vi "Data_Save_summary.vi"(6 "ErrorIndex":i32, 8 "Data in":T1, 11 "AllControls In":T2) -> (2 "data":string[](array[string]), 3 "dup path":path)   [LabVIEW 2017]
uses:
  Ctrls/AllControls.ctl
  Ctrls/CSV_Data.ctl
  Ctrls/PathChoose.ctl
  <vilib>/Utility/file.llb/Write Delimited Spreadsheet (string).vi
  <vilib>/Utility/file.llb/Read Delimited Spreadsheet (string).vi
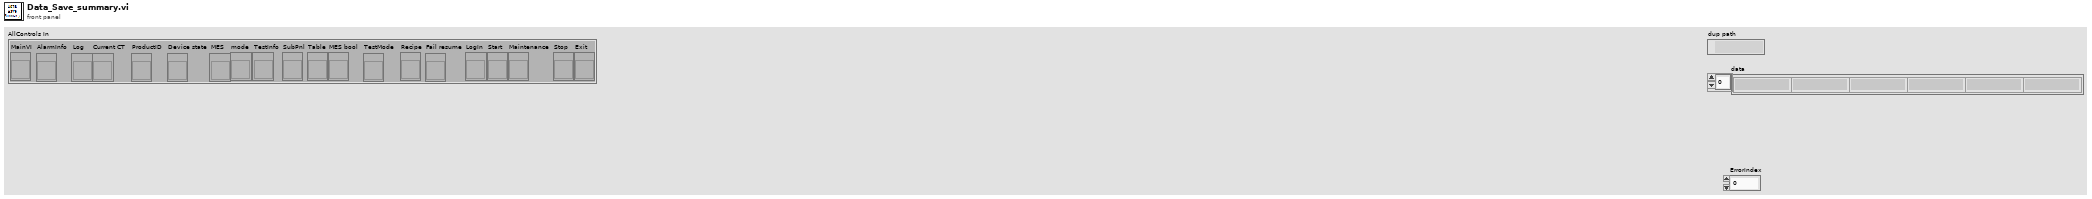
[diagram p1: front panel]
types:
  T1 = typedef "CSV_Data.ctl" = cluster{"Initialisation":cluster{"LMT - Connect UUT (con COM)":string, "LMT - Software Version (rrel)":string, "LMT - Write SKU file (wskuc)":string, "LMT - SKU file name":string, "Connect UUT DDM":string, "Read DDM EOL Timestamp - Mode":string, "Read DDM EOL Timestamp - Timestamp":string, "Read DDM EOL Timestamp - Rig ID":string, "Read DDM EOL Timestamp - Passmark ID":string, "Read DDM EOL Timestamp - Passmark Rev":string, "Software Version before flashing":string, "Read Hardware Serial":string, "UUT DDM SN":string, "Compare DDM SN with MES SN":string, "Backup PCBA Calibration EEPROM Response - CAL":string, "Flash Firmware Version":string, "Check SW Version":string, "Read DDM SW Version after flashing":string, "Set SKU Config":string, "Ready Status":string, "Set Device Mode to EOL":string, "DDM Parameter - Voltage":string, "DDM Parameter - Current":string, "DDM Parameter - Power":string, "DDM Parameter - Speed":string, "DDM Parameter - Pressure":string, "Tester Parameter - Voltage":string, "Tester Parameter - Current":string, "Tester Parameter - Power":string, "Tester Parameter - Ambient Pressure":string, "Tester Parameter - Ambient Temperature":string, "Calculated Parameter - DDM Pressure Corrected":string, "Calculated Parameter - DDM Real Power":string, "Calculated Parameter - Delta V":string}, "BEMF_Calibration":cluster{"Calibration Result - eol_cold_bemf_temp":string, "DDM Ambient Temp":string, "Restriction Plate Diameter":string, "Calibration Result - eol_bemf_mp_cold_coef_a":string, "Calibration Result - eol_bemf_mp_cold_coef_b":string, "Calibration Result - eol_bemf_mp_cold_coef_c":string, "Calibration Result - eol_bemf_lsi_cold_ref_coeffs":string, "Get - Calibration Result - eol_bemf_lsi_speed":string, "Get - Calibration Result - eol_bemf_lsi_integral_0":string, "Calibration Result - eol_bemf_lsi_integral_1":string, "Get - Calibration Result - eol_bemf_lsi_integral_2":string, "Get - Calibration Result - eol_cold_bemf":string, "Get - Calibration Result - eol_cold_bemf_fisf":string, "Finalise Calibration":string, "Compare -Calibration Result - eol_cold_bemf":string, "Compare -Calibration Result - eol_cold_bemf_fisf":string}, "ECO":cluster{"Reset Power Tune":string, "Reset BEMF FISF Calibration":string, "Restriction Plate Diameter":string, "ECO - Stabilisation Time":string, "ECO - DDM Parameter - Voltage":string, "ECO - DDM Parameter - Current":string, "ECO - DDM Parameter - Power":string, "ECO - DDM Parameter - Measured Power":string, "ECO - DDM Parameter - Speed":string, "ECO - DDM Parameter - Pressure":string, "ECO - Tester Parameter - Voltage":string, "ECO - Tester Parameter - Current":string, "ECO - Tester Parameter - Power":string, "ECO - Tester Parameter - Ambient Pressure":string, "ECO - Tester Parameter - Ambient Temperature":string, "ECO - Tester Parameter - Ambient Humidity":string, "ECO - Calculated Parameter - DDM Pressure Corrected":string, "ECO - Calculated Parameter - DDM Real Power":string, "ECO - Calculated Parameter - Delta V":string, "ECO - Calculated Parameter - Flowrate":string, "ECO - Calculated Parameter - Airwatt":string, "ECO - Formula":string, "PT ECO - Power Tune Mode Status":string}, "BOOST":cluster{"Restriction Plate Diameter":string, "BOOST - Stabilisation Time":string, "BOOST - DDM Parameter - Voltage":string, "BOOST - DDM Parameter - Current":string, "BOOST - DDM Parameter - Power":string, "BOOST - DDM Parameter - Measured Power":string, "BOOST - DDM Parameter - Speed":string, "BOOST - DDM Parameter - Pressure":string, "BOOST - Tester Parameter - Voltage":string, "BOOST - Tester Parameter - Current":string, "BOOST - Tester Parameter - Power":string, "BOOST - Tester Parameter - Ambient Pressure":string, "BOOST - Tester Parameter - Ambient Temperature":string, "BOOST - Tester Parameter - Ambient Humidity":string, "BOOST - Calculated Parameter - DDM Pressure Corrected":string, "BOOST - Calculated Parameter - DDM Real Power":string, "BOOST - Calculated Parameter - Delta V":string, "BOOST - Calculated Parameter - Flowrate":string, "BOOST - Calculated Parameter - Airwatt":string, "BOOST - Get AM Presence":string, "Air Muscle Turn Off Status":string, "BOOST - Air Muscle Calculated Parameter - Airwatt B":string, "BOOST - Air Muscle Calculate Airwatt Delta":string, "PT BOOST - Power Tune Mode Status":string, "Finalise Calibration":string, "ECO - Get AW Calibration value":string, "BOOST - Get AW Calibration value":string}, "MAX":cluster{"Restriction Plate Diameter":string, "MAX - Stabilisation Time":string, "Get Average Delta Tmag (LSIdelta_FISFdelta_LSItmag_FISFtmag_IIRtmag)":string, "Get Average Delta Tmag FISF":string, "MAX - DDM Parameter - Voltage":string, "MAX - DDM Parameter - Current":string, "MAX - DDM Parameter - Power":string, "MAX - DDM Parameter - Measured Power":string, "MAX - DDM Parameter - Speed":string, "MAX - DDM Parameter - Pressure":string, "MAX - Tester Parameter - Voltage":string, "MAX - Tester Parameter - Current":string, "MAX - Tester Parameter - Power":string, "MAX - Tester Parameter - Ambient Pressure":string, "MAX - Tester Parameter - Ambient Temperature":string, "MAX - Tester Parameter - Ambient Humidity":string, "MAX - Calculated Parameter - DDM Pressure Corrected":string, "MAX - Calculated Parameter - DDM Real Power":string, "MAX - Calculated Parameter - Delta V":string, "MAX - Calculated Parameter - Flowrate":string, "MAX - Calculated Parameter - Airwatt":string, "MAX_FISF_Check_Average_Delta_Tmag":string, "MAX - FISF - BEMF Finetune Result":string, "MAX tune - Delta P1":string, "MAX tune - Calculated Parameter - Airwatt":string, "Calculate Delta Airwatts - MAX finetune - Delta P2":string, "MAX finetune - DDM Parameter - Voltage":string, "MAX finetune - DDM Parameter - Current":string, "MAX finetune - DDM Parameter - Power":string, "MAX finetune - DDM Parameter - Measured Power":string, "MAX finetune - DDM Parameter - Speed":string, "MAX finetune - DDM Parameter - Pressure":string, "MAX finetune - Tester Parameter - Voltage":string, "MAX finetune - Tester Parameter - Current":string, "MAX finetune - Tester Parameter - Power":string, "MAX finetune - Tester Parameter - Ambient Pressure":string, "MAX finetune - Tester Parameter - Ambient Temperature":string, "MAX finetune - Tester Parameter - Ambient Humidity":string, "MAX finetune - Calculated Parameter - DDM Pressure Corrected":string, "MAX finetune - Calculated Parameter - DDM Real Power":string, "MAX finetune - Calculated Parameter - Delta V":string, "MAX finetune - Calculated Parameter - Flowrate":string, "MAX finetune - Calculated Parameter - Airwatt":string, "Check Derate Result":string, "Delta Tmag FISF":string, "Get Hot BEMF Result":string, "Calculate delta Pressure":string, "Finalise Calibration":string, "Calculate & Check Delta BEMF":string, "Delta P Airwatts Value":string}, "LL":cluster{"DDM Ambient Temp":string, "Restriction Plate Diameter":string, "LL - DDM Parameter - Voltage":string, "LL - DDM Parameter - Current":string, "LL - DDM Parameter - Power":string, "LL - DDM Parameter - Measured Power":string, "LL - DDM Parameter - Speed":string, "LL - DDM Parameter - Pressure":string, "LL - Tester Parameter - Voltage":string, "LL - Tester Parameter - Current":string, "LL - Tester Parameter - Power":string, "LL - DDM Real Power":string, "LL - Calibrate Task Detect LL":string}, "HL":cluster{"HL - DDM Parameter - Voltage":string, "HL - DDM Parameter - Current":string, "HL - DDM Parameter - Power":string, "HL - DDM Parameter - Measured Power":string, "HL - DDM Parameter - Speed":string, "HL - DDM Parameter - Pressure":string, "HL - Tester Parameter - Voltage":string, "HL - Tester Parameter - Current":string, "HL - Tester Parameter - Power":string, "HL - DDM Real Power":string, "HL - Calibrate Task Detect HL":string}, "LH":cluster{"Restriction Plate Diameter":string, "LH - DDM Parameter - Voltage":string, "LH - DDM Parameter - Current":string, "LH - DDM Parameter - Power":string, "LH - DDM Parameter - Measured Power":string, "LH - DDM Parameter - Speed":string, "LH - DDM Parameter - Pressure":string, "LH - Tester Parameter - Voltage":string, "LH - Tester Parameter - Current":string, "LH - Tester Parameter - Power":string, "LH - DDM Real Power":string, "LH - Calibrate Task Detect LH":string}, "HH":cluster{"HH - DDM Parameter - Voltage":string, "HH - DDM Parameter - Current":string, "HH - DDM Parameter - Power":string, "HH - DDM Parameter - Measured Power":string, "HH - DDM Parameter - Speed":string, "HH - DDM Parameter - Pressure":string, "HH - Tester Parameter - Voltage":string, "HH - Tester Parameter - Current":string, "HH - Tester Parameter - Power":string, "HH - DDM Real Power":string, "HH - Calibrate Task Detect HH":string}, "Inlet Blockage Calibration":cluster{"Inlet Blockage Calibration - DDM Parameter - Voltage":string, "Inlet Blockage Calibration - DDM Parameter - Current":string, "Inlet Blockage Calibration - DDM Parameter - Power":string, "Inlet Blockage Calibration - DDM Parameter - Measured Power":string, "Inlet Blockage Calibration - DDM Parameter - Speed":string, "Inlet Blockage Calibration - DDM Parameter - Pressure":string, "Inlet Blockage Calibration - Tester Parameter - Voltage":string, "Inlet Blockage Calibration - Tester Parameter - Current":string, "Inlet Blockage Calibration - Tester Parameter - Power":string, "Inlet Blockage Calibration - DDM Real Power":string, "Calibration Inlet Blockage_E":string, "Finalise Calibration":string, "Get Task Detect LL":string, "Get Task Detect HL":string, "Get Task Detect LH":string, "Get Task Detect HH":string, "Calibration Inlet Blockage":string, "Calibration eol cold bemf temp":string}, "GOOD":cluster{"GOOD UNIT - Clear EEPROM Error Log":string, "GOOD UNIT - Write Product Timestamp - Mode":string, "GOOD UNIT - Write Product Timestamp - Timestamp":string, "GOOD UNIT - Write Product Timestamp - Rig ID":string, "GOOD UNIT - Write Product Timestamp - Passmark ID":string, "GOOD UNIT - Write Product Timestamp - Passmark Rev":string, "GOOD UNIT - Set Device Mode to PROD":string, "GOOD UNIT - Backup PCBA Calibration EEPROM Response":string, "GOOD UNIT - Check Security Bit":string, "GOOD UNIT - Set Calibration Lock":string, "GOOD UNIT - Get_Calibration_Lock":string, "GOOD UNIT - Disconnect UUT":string}, "NG":cluster{"NG UNIT - Read NVM Error":string, "NG UNIT - Set Device Mode to FCT":string, "NG UNIT - Backup PCBA Calibration EEPROM Response - CAL":string, "NG UNIT - Backup PCBA Calibration EEPROM Response - ERROR":string, "NG UNIT - Backup PCBA Calibration EEPROM Response - USAGE":string, "NG UNIT - Disconnect UUT":string}, "SN":string, "Table":string[][], "Count":cluster{"Total":i32, "OK":i32, "NG":i32, "Yield":dbl}, "Start Time":timestamp, "daemon reference":refnum<k5>, "CT":dbl, "Config":string[][], "OK/NG":bool, "Station ID":string, "MES DDM SN":string, "MES PCBA SN":string, "Retest":string, "Lux":string, "Initialisation_Status":cluster{"LMT - Connect UUT (con COM)":string, "LMT - Software Version (rrel)":string, "LMT - Write SKU file (wskuc)":string, "LMT - SKU file name":string, "Connect UUT DDM":string, "Read DDM EOL Timestamp - Mode":string, "Read DDM EOL Timestamp - Timestamp":string, "Read DDM EOL Timestamp - Rig ID":string, "Read DDM EOL Timestamp - Passmark ID":string, "Read DDM EOL Timestamp - Passmark Rev":string, "Software Version before flashing":string, "Read Hardware Serial":string, "UUT DDM SN":string, "Compare DDM SN with MES SN":string, "Backup PCBA Calibration EEPROM Response - CAL":string, "Flash Firmware Version":string, "Check SW Version":string, "Read DDM SW Version after flashing":string, "Set SKU Config":string, "Ready Status":string, "Set Device Mode to EOL":string, "DDM Parameter - Voltage":string, "DDM Parameter - Current":string, "DDM Parameter - Power":string, "DDM Parameter - Speed":string, "DDM Parameter - Pressure":string, "Tester Parameter - Voltage":string, "Tester Parameter - Current":string, "Tester Parameter - Power":string, "Tester Parameter - Ambient Pressure":string, "Tester Parameter - Ambient Temperature":string, "Calculated Parameter - DDM Pressure Corrected":string, "Calculated Parameter - DDM Real Power":string, "Calculated Parameter - Delta V":string}, "BEMF_Calibration_Status":cluster{"Calibration Result - eol_cold_bemf_temp":string, "DDM Ambient Temp":string, "Restriction Plate Diameter":string, "Calibration Result - eol_bemf_mp_cold_coef_a":string, "Calibration Result - eol_bemf_mp_cold_coef_b":string, "Calibration Result - eol_bemf_mp_cold_coef_c":string, "Calibration Result - eol_bemf_lsi_cold_ref_coeffs":string, "Get - Calibration Result - eol_bemf_lsi_speed":string, "Get - Calibration Result - eol_bemf_lsi_integral_0":string, "Calibration Result - eol_bemf_lsi_integral_1":string, "Get - Calibration Result - eol_bemf_lsi_integral_2":string, "Get - Calibration Result - eol_cold_bemf":string, "Get - Calibration Result - eol_cold_bemf_fisf":string, "Finalise Calibration":string, "Compare -Calibration Result - eol_cold_bemf":string, "Compare -Calibration Result - eol_cold_bemf_fisf":string}, "ECO_Status":cluster{"Reset Power Tune":string, "Reset BEMF FISF Calibration":string, "Restriction Plate Diameter":string, "ECO - Stabilisation Time":string, "ECO - DDM Parameter - Voltage":string, "ECO - DDM Parameter - Current":string, "ECO - DDM Parameter - Power":string, "ECO - DDM Parameter - Measured Power":string, "ECO - DDM Parameter - Speed":string, "ECO - DDM Parameter - Pressure":string, "ECO - Tester Parameter - Voltage":string, "ECO - Tester Parameter - Current":string, "ECO - Tester Parameter - Power":string, "ECO - Tester Parameter - Ambient Pressure":string, "ECO - Tester Parameter - Ambient Temperature":string, "ECO - Tester Parameter - Ambient Humidity":string, "ECO - Calculated Parameter - DDM Pressure Corrected":string, "ECO - Calculated Parameter - DDM Real Power":string, "ECO - Calculated Parameter - Delta V":string, "ECO - Calculated Parameter - Flowrate":string, "ECO - Calculated Parameter - Airwatt":string, "ECO - Formula":string, "PT ECO - Power Tune Mode Status":string}, "BOOST_Status":cluster{"Restriction Plate Diameter":string, "BOOST - Stabilisation Time":string, "BOOST - DDM Parameter - Voltage":string, "BOOST - DDM Parameter - Current":string, "BOOST - DDM Parameter - Power":string, "BOOST - DDM Parameter - Measured Power":string, "BOOST - DDM Parameter - Speed":string, "BOOST - DDM Parameter - Pressure":string, "BOOST - Tester Parameter - Voltage":string, "BOOST - Tester Parameter - Current":string, "BOOST - Tester Parameter - Power":string, "BOOST - Tester Parameter - Ambient Pressure":string, "BOOST - Tester Parameter - Ambient Temperature":string, "BOOST - Tester Parameter - Ambient Humidity":string, "BOOST - Calculated Parameter - DDM Pressure Corrected":string, "BOOST - Calculated Parameter - DDM Real Power":string, "BOOST - Calculated Parameter - Delta V":string, "BOOST - Calculated Parameter - Flowrate":string, "BOOST - Calculated Parameter - Airwatt":string, "BOOST - Get AM Presence":string, "Air Muscle Turn Off Status":string, "BOOST - Air Muscle Calculated Parameter - Airwatt B":string, "BOOST - Air Muscle Calculate Airwatt Delta":string, "PT BOOST - Power Tune Mode Status":string, "Finalise Calibration":string, "ECO - Get AW Calibration value":string, "BOOST - Get AW Calibration value":string}, "MAX_Status":cluster{"Restriction Plate Diameter":string, "MAX - Stabilisation Time":string, "Get Average Delta Tmag (LSIdelta_FISFdelta_LSItmag_FISFtmag_IIRtmag)":string, "Get Average Delta Tmag FISF":string, "MAX - DDM Parameter - Voltage":string, "MAX - DDM Parameter - Current":string, "MAX - DDM Parameter - Power":string, "MAX - DDM Parameter - Measured Power":string, "MAX - DDM Parameter - Speed":string, "MAX - DDM Parameter - Pressure":string, "MAX - Tester Parameter - Voltage":string, "MAX - Tester Parameter - Current":string, "MAX - Tester Parameter - Power":string, "MAX - Tester Parameter - Ambient Pressure":string, "MAX - Tester Parameter - Ambient Temperature":string, "MAX - Tester Parameter - Ambient Humidity":string, "MAX - Calculated Parameter - DDM Pressure Corrected":string, "MAX - Calculated Parameter - DDM Real Power":string, "MAX - Calculated Parameter - Delta V":string, "MAX - Calculated Parameter - Flowrate":string, "MAX - Calculated Parameter - Airwatt":string, "MAX_FISF_Check_Average_Delta_Tmag":string, "MAX - FISF - BEMF Finetune Result":string, "MAX tune - Delta P1":string, "MAX tune - Calculated Parameter - Airwatt":string, "Calculate Delta Airwatts - MAX finetune - Delta P2":string, "MAX finetune - DDM Parameter - Voltage":string, "MAX finetune - DDM Parameter - Current":string, "MAX finetune - DDM Parameter - Power":string, "MAX finetune - DDM Parameter - Measured Power":string, "MAX finetune - DDM Parameter - Speed":string, "MAX finetune - DDM Parameter - Pressure":string, "MAX finetune - Tester Parameter - Voltage":string, "MAX finetune - Tester Parameter - Current":string, "MAX finetune - Tester Parameter - Power":string, "MAX finetune - Tester Parameter - Ambient Pressure":string, "MAX finetune - Tester Parameter - Ambient Temperature":string, "MAX finetune - Tester Parameter - Ambient Humidity":string, "MAX finetune - Calculated Parameter - DDM Pressure Corrected":string, "MAX finetune - Calculated Parameter - DDM Real Power":string, "MAX finetune - Calculated Parameter - Delta V":string, "MAX finetune - Calculated Parameter - Flowrate":string, "MAX finetune - Calculated Parameter - Airwatt":string, "Check Derate Result":string, "Delta Tmag FISF":string, "Get Hot BEMF Result":string, "Calculate delta Pressure":string, "Finalise Calibration":string, "Calculate & Check Delta BEMF":string, "Delta P Airwatts Value":string}, "LL_Status":cluster{"DDM Ambient Temp":string, "Restriction Plate Diameter":string, "LL - DDM Parameter - Voltage":string, "LL - DDM Parameter - Current":string, "LL - DDM Parameter - Power":string, "LL - DDM Parameter - Measured Power":string, "LL - DDM Parameter - Speed":string, "LL - DDM Parameter - Pressure":string, "LL - Tester Parameter - Voltage":string, "LL - Tester Parameter - Current":string, "LL - Tester Parameter - Power":string, "LL - DDM Real Power":string, "LL - Calibrate Task Detect LL":string}, "HL_Status":cluster{"HL - DDM Parameter - Voltage":string, "HL - DDM Parameter - Current":string, "HL - DDM Parameter - Power":string, "HL - DDM Parameter - Measured Power":string, "HL - DDM Parameter - Speed":string, "HL - DDM Parameter - Pressure":string, "HL - Tester Parameter - Voltage":string, "HL - Tester Parameter - Current":string, "HL - Tester Parameter - Power":string, "HL - DDM Real Power":string, "HL - Calibrate Task Detect HL":string}, "LH_Status":cluster{"Restriction Plate Diameter":string, "LH - DDM Parameter - Voltage":string, "LH - DDM Parameter - Current":string, "LH - DDM Parameter - Power":string, "LH - DDM Parameter - Measured Power":string, "LH - DDM Parameter - Speed":string, "LH - DDM Parameter - Pressure":string, "LH - Tester Parameter - Voltage":string, "LH - Tester Parameter - Current":string, "LH - Tester Parameter - Power":string, "LH - DDM Real Power":string, "LH - Calibrate Task Detect LH":string}, "HH_Status":cluster{"HH - DDM Parameter - Voltage":string, "HH - DDM Parameter - Current":string, "HH - DDM Parameter - Power":string, "HH - DDM Parameter - Measured Power":string, "HH - DDM Parameter - Speed":string, "HH - DDM Parameter - Pressure":string, "HH - Tester Parameter - Voltage":string, "HH - Tester Parameter - Current":string, "HH - Tester Parameter - Power":string, "HH - DDM Real Power":string, "HH - Calibrate Task Detect HH":string}, "Inlet Blockage Calibration_Status":cluster{"Inlet Blockage Calibration - DDM Parameter - Voltage":string, "Inlet Blockage Calibration - DDM Parameter - Current":string, "Inlet Blockage Calibration - DDM Parameter - Power":string, "Inlet Blockage Calibration - DDM Parameter - Measured Power":string, "Inlet Blockage Calibration - DDM Parameter - Speed":string, "Inlet Blockage Calibration - DDM Parameter - Pressure":string, "Inlet Blockage Calibration - Tester Parameter - Voltage":string, "Inlet Blockage Calibration - Tester Parameter - Current":string, "Inlet Blockage Calibration - Tester Parameter - Power":string, "Inlet Blockage Calibration - DDM Real Power":string, "Calibration Inlet Blockage_E":string, "Finalise Calibration":string, "Get Task Detect LL":string, "Get Task Detect HL":string, "Get Task Detect LH":string, "Get Task Detect HH":string, "Calibration Inlet Blockage":string, "Calibration eol cold bemf temp":string}, "GOOD_Status":cluster{"GOOD UNIT - Clear EEPROM Error Log":string, "GOOD UNIT - Write Product Timestamp - Mode":string, "GOOD UNIT - Write Product Timestamp - Timestamp":string, "GOOD UNIT - Write Product Timestamp - Rig ID":string, "GOOD UNIT - Write Product Timestamp - Passmark ID":string, "GOOD UNIT - Write Product Timestamp - Passmark Rev":string, "GOOD UNIT - Set Device Mode to PROD":string, "GOOD UNIT - Backup PCBA Calibration EEPROM Response":string, "GOOD UNIT - Check Security Bit":string, "GOOD UNIT - Set Calibration Lock":string, "GOOD UNIT - Get_Calibration_Lock":string, "GOOD UNIT - Disconnect UUT":string}, "NG_Status":cluster{"NG UNIT - Read NVM Error":string, "NG UNIT - Set Device Mode to FCT":string, "NG UNIT - Backup PCBA Calibration EEPROM Response - CAL":string, "NG UNIT - Backup PCBA Calibration EEPROM Response - ERROR":string, "NG UNIT - Backup PCBA Calibration EEPROM Response - USAGE":string, "NG UNIT - Disconnect UUT":string}, "SKU":string, "Plate_Diameter":string, "Alarm":string}
  T2 = typedef "AllControls.ctl" = cluster{"MainVI":refnum<vi>, "AlarmInfo":refnum<vi>, "Log":refnum<vi>, "Current CT":refnum<vi>, "ProductID":refnum<vi>, "Device state":refnum<vi>, "MES":refnum<vi>, "mode":refnum<vi>, "TestInfo":refnum<vi>, "SubPnl":refnum<vi>, "Table":refnum<vi>, "MES bool":refnum<vi>, "TestMode":refnum<vi>, "Recipe":refnum<vi>, "Fail resume":refnum<vi>, "LogIn":refnum<vi>, "Start":refnum<vi>, "Maintenance":refnum<vi>, "Stop":refnum<vi>, "Exit":refnum<vi>}
  T3 = typedef "PathChoose.ctl" = enum16{"OperatorLog", "AutoRunLog", "AlmLog", "TestData", "AllTestData", "backup_nvm", "backup_before_flashing"}
  T4 = typedef "TesterInfo.ctl" = cluster{"Station Name":string, "Station Code":string, "ES NO.":string, "Tester ID":string, "PassMark Revision":string, "Rig ID":string, "Deamon_vision":string, "Project Name":string, "FFTesterPath":path, "Enable_User":bool, "Mode":enum16{"682"}, "MES":bool}
  T5 = typedef "HD Config.ctl" = cluster{" PC":cluster{"PC Address":u8[], "PC Port":i32}, "FCO":cluster{"COM":refnum<visa-resource-name>, "Baudrate":u32}, "DC Power ":cluster{"COM":refnum<visa-resource-name>, "Baudrate":u32}, "PW3336":cluster{"COM":refnum<visa-resource-name>, "Baudrate":u32}, "Lefoo":cluster{"COM":refnum<visa-resource-name>, "Baudrate":u32}, "Tempt&Hum":cluster{"COM":refnum<visa-resource-name>, "Baudrate":u32}, "DIPC":cluster{"COM":refnum<visa-resource-name>}, "Daemon":cluster{"IP Address":string, "Port":u16, "Retry":u16}, "URAT":cluster{"COM":refnum<visa-resource-name>, "Baudrate":u32}, "Fail_resume_mode":bool, "GRR":bool}
  T6 = enum16{"open", "replace", "create", "open or create", "replace or create", "replace or create with confirmation"}
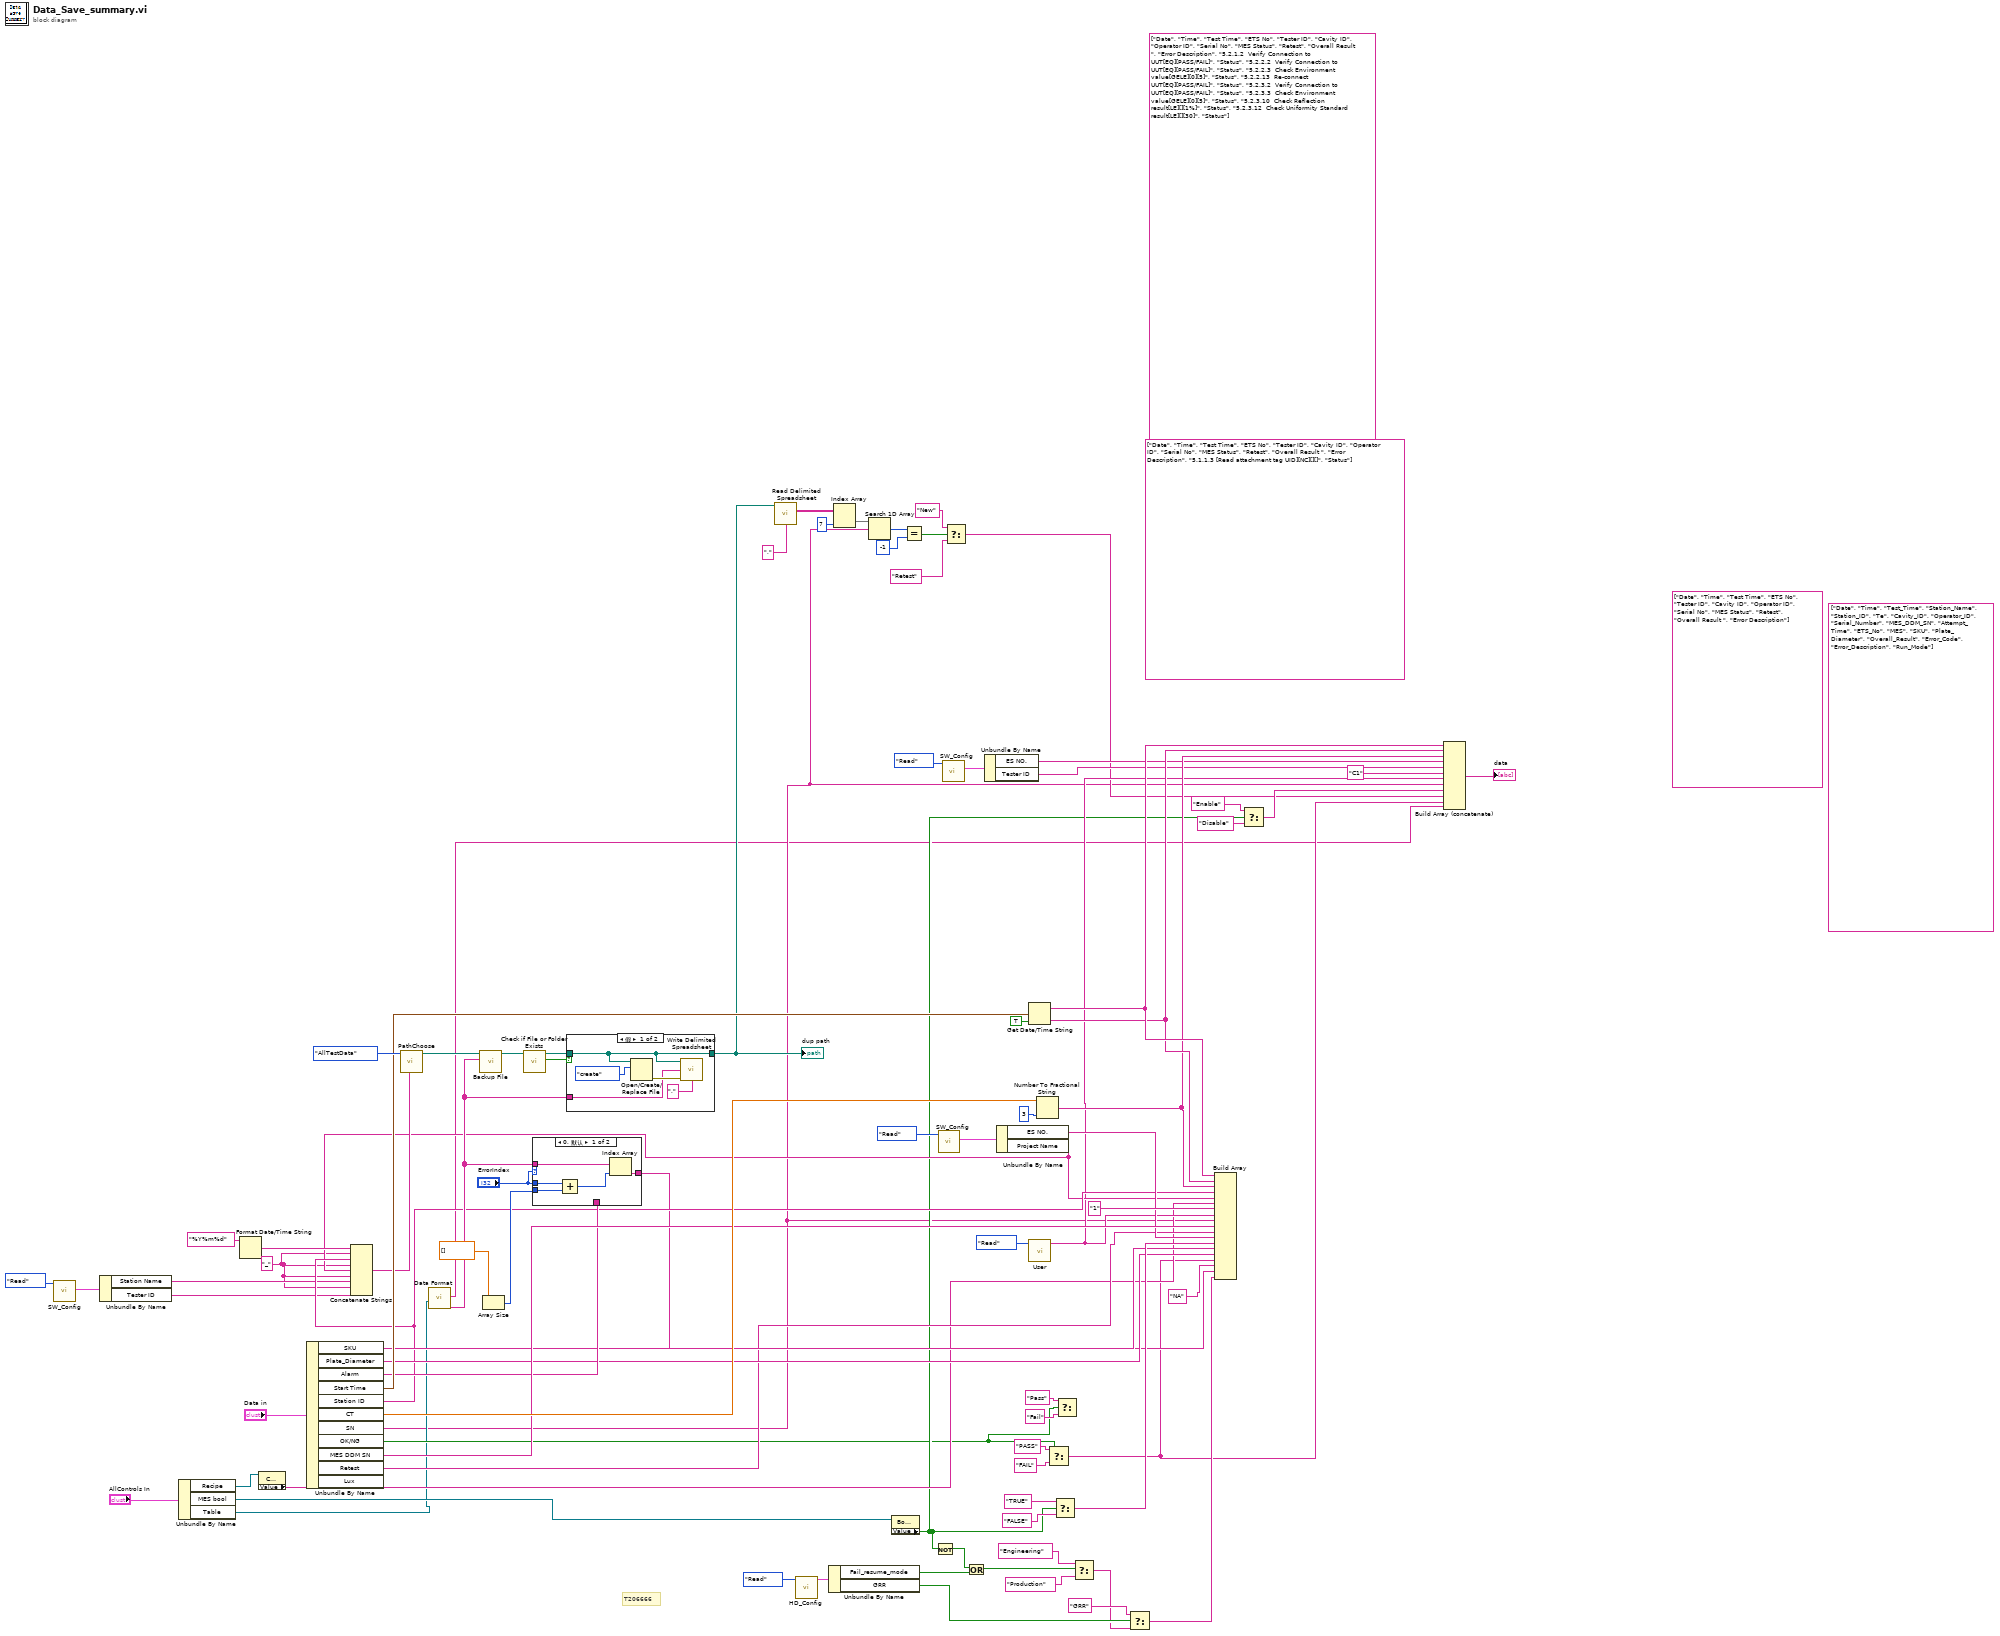
[diagram p0: block diagram]
diagram:
  (unwired) string[] ["Date", "Time", "Test Time", "ETS No", "Tester ID", "Cavity ID", "Operator ID", "Serial No", "MES Status", "Retest", "Overall Result ", "Error Description", "5.2.1.2  Verify Connection to UUT[EQ][PASS/FAIL]", "Status", "5.2.2.2  Verify Connection to UUT[EQ][PASS/FAIL]", "Status", "5.2.2.3  Check Environment value[GELE][0][5]", "Status", "5.2.2.13  Re-connect UUT[EQ][PASS/FAIL]", "Status", "5.2.3.2  Verify Connection to UUT[EQ][PASS/FAIL]", "Status", "5.2.3.3  Check Environment value[GELE][0][5]", "Status", "5.2.3.10  Check Reflection result[LE][][1%]", "Status", "5.2.3.12  Check Uniformity Standard result[LE][][30]", "Status"] ("title")
  (unwired) string[] ["Date", "Time", "Test Time", "ETS No", "Tester ID", "Cavity ID", "Operator ID", "Serial No", "MES Status", "Retest", "Overall Result ", "Error Description", "5.1.1.3 [Read attachment tag UID][NC][][]", "Status"] ("title")
  (unwired) string[] ["Date", "Time", "Test Time", "ETS No", "Tester ID", "Cavity ID", "Operator ID", "Serial No", "MES Status", "Retest", "Overall Result ", "Error Description"] ("title")
  w23 = "_" ("字符串")
  (unwired) string[] ["Date", "Time", "Test_Time", "Station_Name", "Station_ID", "Te", "Cavity_ID", "Operator_ID", "Serial_Number", "MES_DDM_SN", "Attempt_Time", "ETS_No", "MES", "SKU", "Plate_Diameter", "Overall_Result", "Error_Code", "Error_Description", "Run_Mode"]
  # "T206666"
  n1 = call "SW_Config.vi"("Step"=enum16{"Initial", "Write", "Read"}."Read") -> ("SW Config out"=w25:T4)  [unwired: 9 in, 1 out]
  n2 = Unbundle By Name(w25) -> ("Station Name"=w24:string, "Tester ID"=w22:string)
  n3 = Unbundle By Name("AllControls In") -> ("Recipe"=w55:refnum<vi>, "MES bool"=w75:refnum<vi>, "Table"=w15:refnum<vi>)
  n4 = Format Date/Time String(time format string (%c)="%Y%m%d") -> (date/time string=w46:string)  [unwired: 2 in]
  n5 = property class="CmbBox"(reference=w55) -> ("Value"=w21:string)  [unwired: 1 in, 2 out]
  n6 = Unbundle By Name("Data in") -> ("SKU"=w49:string, "Plate_Diameter"=w48:string, "Alarm"=w50:string, "Start Time"=w53:timestamp, "Station ID"=w44:string, "CT"=w77:dbl, "SN"=w2:string, "OK/NG"=w16:bool, "MES DDM SN"=w63:string, "Retest"=w27:string)  [unwired: 1 out]
  n7 = call "Data Format.vi"("Table"=w15) -> ("title"=w54:string[], "Data"=w1:string[])  [unwired: 9 in]
  n8 = Array Size(array=dbl[] []) -> (size(s)=w51:i32)
  n9 = case shown="0, 默认" "ErrorIndex" {
    tunnel: w54 -> [w93 _]
    tunnel: "ErrorIndex" -> [w92 _]
    tunnel: [w90 w94] -> w29
    tunnel: w51 -> [w89 _]
    tunnel: w50 -> [_ w94]
    frame 0, Default {
      n10 = Add(x=w92, y=w89) -> (x+y=w91:i32)
      n11 = Index Array(array=w93, index=w91) -> (element=w90:string)
    }
    frame -1 {
    }
  }
  n12 = call "HD_Config.vi"("Step"=enum16{"Initial", "Write", "Read"}."Read") -> ("HD Config out"=w72:T5)  [unwired: 9 in, 1 out]
  n13 = Unbundle By Name(w72) -> ("Fail_resume_mode"=w66:bool, "GRR"=w62:bool)
  n14 = property class="Bool (严格)"(reference=w75) -> ("Value"=w20:bool)  [unwired: 1 in, 2 out]
  n15 = Not(x=w20) -> (.not. x?=w64:bool)
  n16 = call "SW_Config.vi"("Step"=enum16{"Initial", "Write", "Read"}."Read") -> ("SW Config out"=w88:T4)  [unwired: 9 in, 1 out]
  n17 = call "SW_Config.vi"("Step"=enum16{"Initial", "Write", "Read"}."Read") -> ("SW Config out"=w38:T4)  [unwired: 9 in, 1 out]
  n18 = Or(x=w64, y=w66) -> (x .or. y?=w65:bool)
  n19 = Unbundle By Name(w38) -> ("ES NO."=w37:string, "Tester ID"=w36:string)
  n20 = Unbundle By Name(w88) -> ("ES NO."=w57:string, "Project Name"=w43:string)
  n21 = Concatenate Strings(w46, w23, w44, w23, w43, w23, w24, w23, w22) -> (w45:string)
  n22 = call "PathChoose.vi"("csv Name"=w45, 11:PathChoose."AllTestData") -> ("Path_Out"=w69:path)  [unwired: 9 in]
  n23 = call "Backup File.vi"("列首字符串"=w54, "path"=w69) -> ("path 2"=w68:path)  [unwired: 9 in]
  n24 = call <vilib>:"Check if File or Folder Exists.vi"("path"=w68) -> ("file or folder exists?"=w82:bool, "dup path"=w81:path)  [unwired: 8 in, 1 out]
  n25 = case shown="假" w82 {
    tunnel: w81 -> [w97 w100]
    tunnel: [w97 w100] -> w13
    tunnel: w54 -> [w95 _]
    frame False {
      n26 = Open/Create/Replace File(file path (use dialog)=w97, operation (0:open)=T6."create") -> (error out=w96:errorcluster)  [unwired: 4 in, 2 out]
      n27 = call-poly <vilib>:"Write Delimited Spreadsheet.vi"("file path (dialog if empty)"=w97, "1D data"=w95, "error in (no error)"=w96, "delimiter (\\t)"="," ("delimiter (\\t)")) -> ()  [unwired: 10 in, 2 out]
    }
    frame True {
    }
  }
  "dup path" <- w13
  n28 = call-poly <vilib>:"Read Delimited Spreadsheet.vi"("file path (dialog if empty)"=w13, "delimiter (\\t)"="," ("delimiter (\\t)")) -> ("all rows"=w11:string[][])  [unwired: 8 in, 5 out]
  n29 = Index Array(array=w11, index (col)=7 ("disabled index (col)")) -> (element=w9:string[])  [unwired: 1 in]
  n30 = Search 1D Array(1D array=w9, element=w2) -> (index of element=w8:i32)  [unwired: 1 in]
  n31 = Equal?(x=w8, y=-1) -> (x = y?=w6:bool)
  n32 = Select(t="New", s=w6, f="Retest") -> (s? t:f=w3:string)
  n33 = Get Date/Time String(seconds (now)=w53, want seconds? (F)=TRUE ("需要秒？(F)")) -> (date string=w42:string, time string=w41:string)  [unwired: 1 in]
  n34 = call "User.vi"("Step"=enum16{"Initial", "Write", "Read"}."Read") -> ("User out"=w34:string)  [unwired: 9 in, 1 out]
  n35 = Number To Fractional String(number=w77, precision (6)=i16 3 ("精度(6)")) -> (F-format string=w40:string)  [unwired: 2 in]
  n36 = Select(t="PASS" ("真字符串"), s=w16, f="FAIL" ("假字符串")) -> (s? t:f=w19:string)
  n37 = Select(t="TRUE" ("真字符串"), s=w20, f="FALSE" ("假字符串")) -> (s? t:f=w56:string)
  n38 = Select(t="Pass" ("真字符串"), s=w16, f="Fail" ("假字符串")) -> ()  [unwired: 1 out]
  n39 = Select(t="Engineering", s=w65, f="Production") -> (s? t:f=w60:string)
  n40 = Select(t="GRR", s=w62, f=w60) -> (s? t:f=w59:string)
  n41 = Build Array(w42, w41, w40, w44, w43, w21, "1" ("Cavity ID_L"), w34, w2, w63, w27, w57, w56, w49, w48, w19, "NA" ("element"), w29, w59) -> ()  [unwired: 1 out]
  n42 = Select(t="Enable" ("element"), s=w20, f="Disable") -> (s? t:f=w31:string)
  n43 = Build Array (concatenate)(w42, w41, w40, w37, w36, "C1" ("element"), w34, w2, w31, w3, w19, w1) -> (→"data":string[])
